vi "test_save_data.vi"() -> ()   [LabVIEW 2020]
panel:
  out "size(s)":i32
  out "Y":i32
  out "X":i32
  out "x+y":i32
  in  "stop":bool
  in  "Array":dbl[](array[numeric])
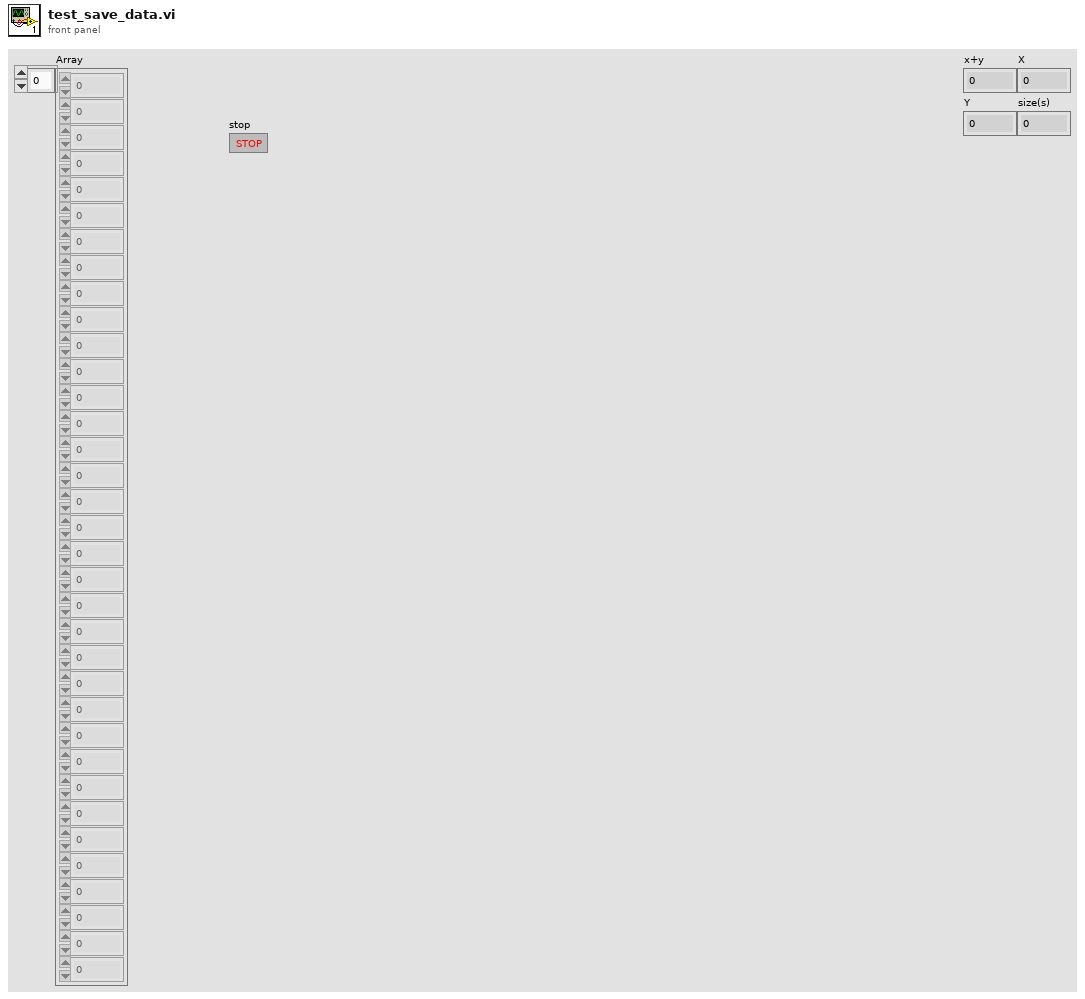
[diagram p1: front panel]
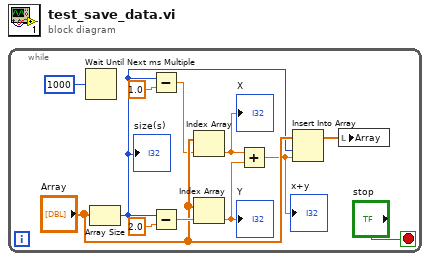
[diagram p0: block diagram]
diagram:
  n1 = while {
    stop <- "stop" stop-if-true
    n2 = Wait Until Next ms Multiple(millisecond multiple=u32 1000) -> ()  [unwired: 1 out]
    n3 = Array Size(array="Array") -> (size(s)=w2:i32)
    "size(s)" <- w2
    n4 = Subtract(x=w2, y=1.0) -> (x-y=w1:dbl)
    n5 = Subtract(x=w2, y=2.0) -> (x-y=w8:dbl)
    n6 = Index Array(array="Array", index=w1) -> (element=w6:dbl)
    "X" <- w6
    n7 = Index Array(array="Array", index=w8) -> (element=w5:dbl)
    "Y" <- w5
    n8 = Add(x=w6, y=w5) -> (x+y=w4:dbl)
    "x+y" <- w4
    n9 = Insert Into Array(array="Array", index=w2, new element=w4) -> (w10:dbl[])
    n10 = local write "Array"(w10) -> ()
  }
